vi "LoadTrafficLightsQueue.vi"(0 "Queue Ref in":refnum<queue>, 2 "Walk":bool) -> ()   [LabVIEW 2012]
doc: "Used to Enqueue the Walk Element when Walk button has been pressed. Uses a Queue Reference to efficiently read the address of Red State, Enqueues rest of elements and places Walk State at the front of the Queue."
uses:
  Controls/Traffic Light States (with Walk State).ctl
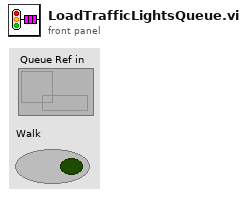
[diagram p1: front panel]
types:
  T1 = typedef "Traffic Light States (with Walk State).ctl" = enum16{"Red", "RedAmber", "Green", "Amber", "Walk"}
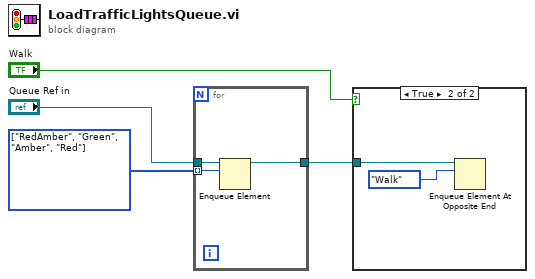
[diagram p0: block diagram]
diagram:
  w2 = T1[] [enum."RedAmber", enum."Green", enum."Amber", enum."Red"] items=["Red", "RedAmber", "Green", "Amber", "Walk"]
  n1 = for {
    tunnel: w2 -> [w7] mode=indexing
    tunnel: "Queue Ref in" -> [w6]
    tunnel: [w5] -> w3
    n2 = Enqueue Element(queue=w6, element=w7) -> (queue out=w5:refnum<queue>)  [unwired: 2 in, 2 out]
  }
  n3 = case "Walk Tunnel\nWalk Tunnel" shown="True" "Walk" {
    tunnel: w3 -> [_ w9]
    frame False {
    }
    frame True {
      n4 = Enqueue Element At Opposite End(queue=w9, element=Traffic_Light_States_(with_Walk_State)."Walk") -> ()  [unwired: 2 in, 3 out]
    }
  }
